vi "sub_deg_to_rad.vi"(11 "deg in":dbl format="%.1f") -> (3 "rad out":dbl format="%.1f")   [LabVIEW 2019]
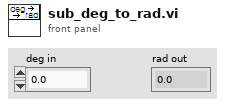
[diagram p1: front panel]
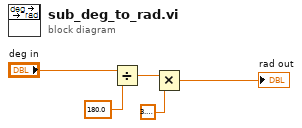
[diagram p0: block diagram]
diagram:
  n1 = Divide(x="deg in", y=180.0) -> (x/y=w1:dbl)
  n2 = Multiply(x=w1, y=3.141592653589793) -> (x*y=→"rad out":dbl)
